vi "RUN 01 reset arms.vi"   [LabVIEW 2016]
types:
  T1 = typedef "LVHSConnector.ctl" = refnum<class "BrickReference.lvclass">
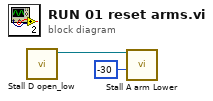
[diagram p0: block diagram]
diagram:
  n1 = call "Stall D open_low.vi"() -> ("NXT/EV3"=w2:T1)  [unwired: 11 in]
  n2 = call "Stall A arm Lower.vi"("Power"=i8 -30, "NXT/EV3"=w2) -> ()  [unwired: 9 in, 1 out]
